vi "waitArmForBusy.vi"(0 "base":bool) -> ()   [LabVIEW 2018]
uses:
  ARM angles.vi
panel:
  out "Numeric":i16
  out "busy 2":bool
  out "busy 1":bool
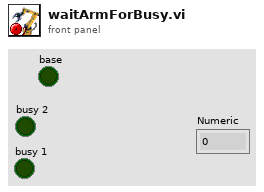
[diagram p1: front panel]
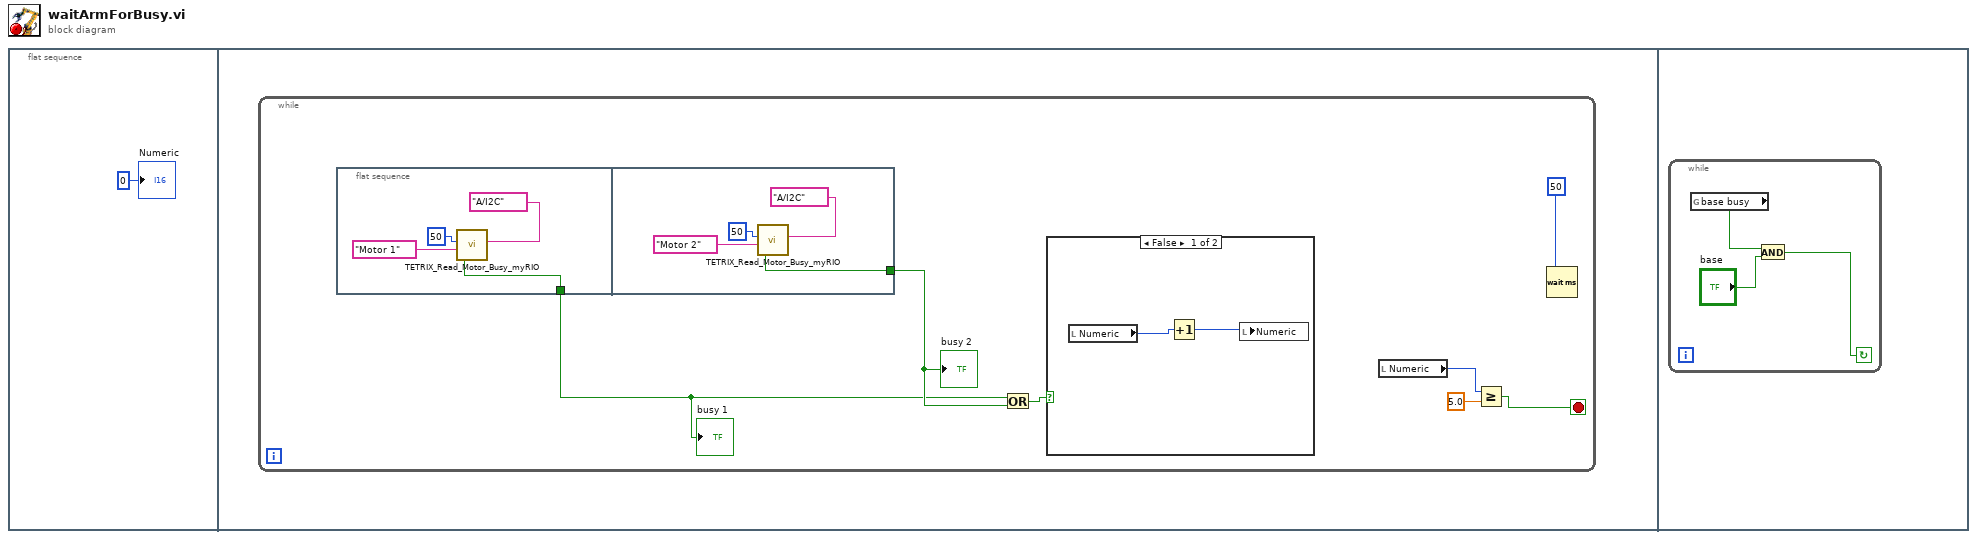
[diagram p0: block diagram]
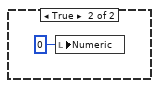
[diagram p2: hidden frame]
diagram:
  n1 = flat-sequence {
    frame #0 {
      "Numeric" <- i16 0 ("Numeric")
    }
    frame #1 {
      n2 = while {
        stop <- w2 stop-if-true
        n3 = flat-sequence {
          tunnel: [w12] -> w7
          tunnel: [w16] -> w8
          frame #0 {
            n4 = call <vilib>:"TETRIX_Read_Motor_Busy_myRIO.vi"("myRIO MXP Port A/B"=tag "A/I2C", "Select Channel"="Motor 1", "Controller ID#  (I2C Address)"=u8 50) -> ("Motor Busy?"=w12:bool)  [unwired: 3 in, 1 out]
          }
          frame #1 {
            n5 = call <vilib>:"TETRIX_Read_Motor_Busy_myRIO.vi"("myRIO MXP Port A/B"=tag "A/I2C", "Select Channel"="Motor 2", "Controller ID#  (I2C Address)"=u8 50) -> ("Motor Busy?"=w16:bool)  [unwired: 3 in, 1 out]
          }
        }
        n6 = Or(x=w7, y=w8) -> (x .or. y?=w5:bool)
        n7 = case shown="False" w5 {
          frame False {
            n8 = local read "Numeric"() -> (w10:i16)
            n9 = Increment(x=w10) -> (x+1=w9:i16)
            n10 = local write "Numeric"(w9) -> ()
          }
          frame True {
            n11 = local write "Numeric"(i16 0 ("Numeric")) -> ()
          }
        }
        n12 = local read "Numeric"() -> (w3:i16)
        n13 = Greater Or Equal?(x=w3, y=5.0) -> (x >= y?=w2:bool)
        n14 = Wait (ms)(milliseconds to wait=u32 50) -> ()  [unwired: 1 out]
        "busy 2" <- w8
        "busy 1" <- w7
      }
    }
    frame #2 {
      n15 = while {
        stop <- w20 continue-if-true
        n16 = global read "ARM angles.vi" "base busy"() -> (w22:bool)
        n17 = And(x=w22, y="base") -> (x .and. y?=w20:bool)
      }
    }
  }
